vi "积分器_采样参数_波形拆解测试.vi"() -> ()   [LabVIEW 2018]
uses:
  <vilib>/measure/NI_MABase.lvlib
  <vilib>/Analysis/NI_AALPro.lvlib
panel:
  out "积分信号":waveform(dbl)(graph)
  out "采样参数（采样频率fs，采样数）":cluster{dbl, dbl} {"?" format="%#_6f"; "?" format="%#_6f"}
  out "载波信号":waveform(dbl)(graph)
  out "已调信号":waveform(dbl)(graph)
  in  "kf(Hz/V)":dbl=50000.0
  in  "An(V)":dbl=0.02
  in  "调制信号":cluster{"fm(Hz)":dbl, "Am(V)":dbl}={"fm(Hz)"=5000.0, "Am(V)"=1.0}
  in  "载波信号":cluster{"fc(Hz)":dbl, "Ac(V)":dbl}={"fc(Hz)"=150000.0, "Ac(V)"=1.0}
  # "要显示n个周期的调制信号波形，则采样数N=n*fs/fm"
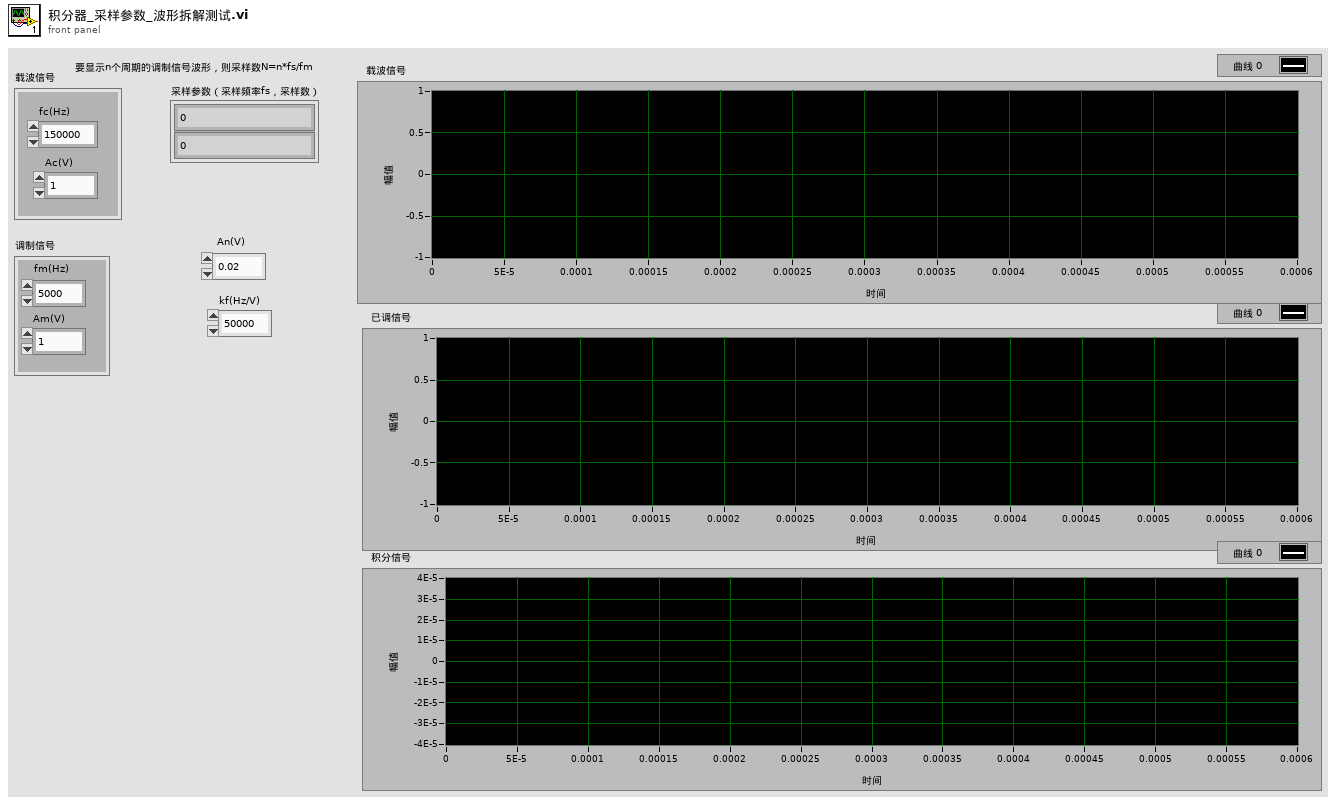
[diagram p1: front panel]
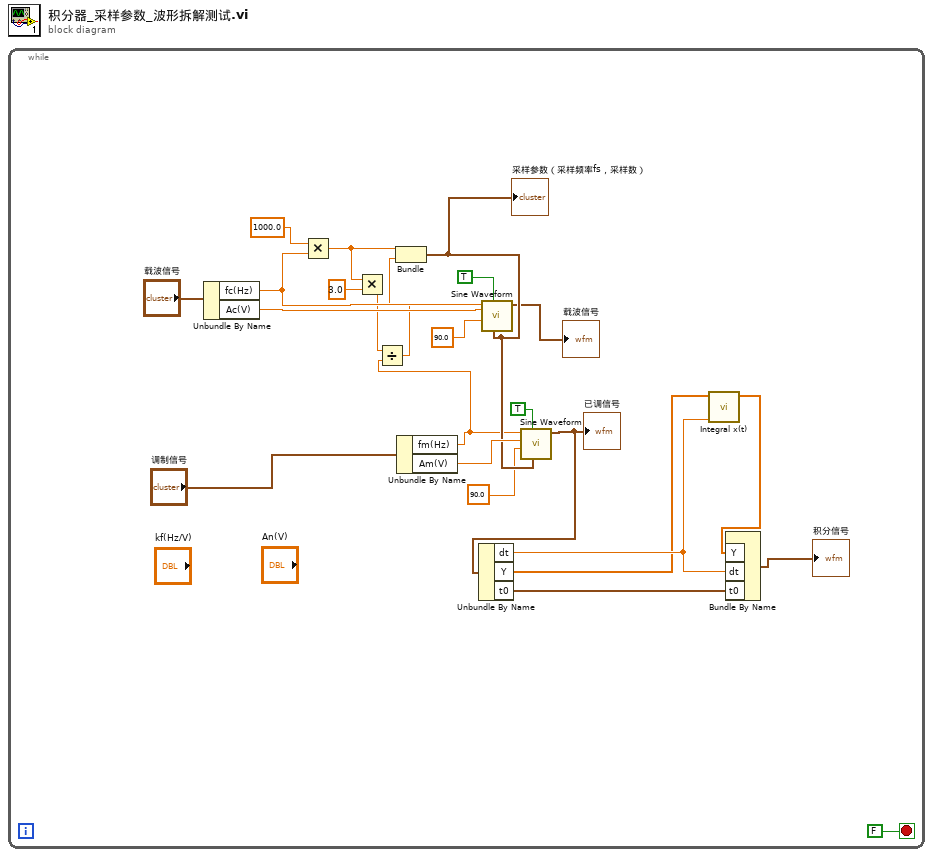
[diagram p0: block diagram]
diagram:
  n1 = while {
    stop <- FALSE stop-if-true
    n2 = Unbundle By Name("载波信号") -> ("fc(Hz)"=w20:dbl, "Ac(V)"=w19:dbl)
    n3 = Multiply(x=1000.0, y=w20) -> (x*y=w10:dbl)
    n4 = Multiply(x=w10, y=3.0) -> (x*y=w9:dbl)
    n5 = Unbundle By Name("调制信号") -> ("fm(Hz)"=w8:dbl, "Am(V)"=w18:dbl)
    n6 = Divide(x=w9, y=w8) -> (x/y=w7:dbl)
    n7 = Bundle(w10, w7) -> (w17:cluster{dbl, dbl})  [unwired: 1 in]
    "采样参数（采样频率fs，采样数）" <- w17
    n8 = call <vilib>:"Sine Waveform.vi"("sampling info"=w17, "reset signal"=TRUE, "phase"=90.0, "amplitude"=w19, "frequency"=w20) -> ("signal out"=→"载波信号":waveform(dbl))  [unwired: 5 in, 1 out]
    n9 = call <vilib>:"Sine Waveform.vi"("sampling info"=w17, "reset signal"=TRUE, "phase"=90.0, "amplitude"=w18, "frequency"=w8) -> ("signal out"=w6:waveform(dbl))  [unwired: 5 in, 1 out]
    "已调信号" <- w6
    n10 = Unbundle By Name(w6) -> ("dt"=w15:dbl, "Y"=w11:dbl[], "t0"=w5:timestamp)
    n11 = call <vilib>:"Integral x(t).vi"("dt"=w15, "X"=w11) -> ("Integral X"=w14:dbl[])  [unwired: 8 in, 1 out]
    n12 = Bundle By Name("Y"=w14, "dt"=w15, "t0"=w5) -> (→"积分信号":waveform(dbl))  [unwired: 1 in]
  }
